vi "DFD M-Band Filter Bank Decomposition with State (Wfm).vi"(6 "state in":cluster{"state ":dbl[]}[](array[cluster]), 7 "t0":timestamp, 8 "error in (no error)":errorcluster, 9 "init?":bool, 10 "analysis bank":T1={"mBank_Filters"=[], " mBank_#Bands"=2, "mBank_ProcMethod"=enum."General", "mBank_Coeffs"=[], "mBank_Gain"=1.0, "mBank_Type"=0} {"mBank_Type" items=["Uniform", "Non-Uniform"]; "mBank_Filters"."mMRate_SumWl" min=1 max=32 step=1; "mBank_Filters"."mMRate_InputIwl" min=1 max=32 step=1; "mBank_Filters"."mMRate_GainWl" min=1 max=32 step=1; "mBank_Filters"."mMRate_OutputWl" min=1 max=32 step=1; "mBank_Filters"."mMRate_InputWl" min=1 max=32 step=1; "mBank_Filters"."mMRate_CoefWl" min=1 max=32 step=1; "mBank_Filters"."mMRate_Mode" items=["Default"=-1, "No Rate Change"=0, "Interpolation"=1, "Decimation"=2, "Interpolated"=3, "Rational"=4]}, 11 "x":waveform(dbl)={"t0"=timestamp(0 s since 1904-01-01), "dt"=0.0, "Y"=[]}) -> (0 "error out":errorcluster, 3 "M bands":waveform(dbl)[](array[waveform]), 4 "state out":cluster{"state ":dbl[]}[](array[cluster]), 5 "tf":timestamp)   [LabVIEW 2017, in "NI_DigFilter_FilterBank.lvlib"]
doc: "Filters the input waveform <B>x</B> using an M-band analysis bank specified by <B>analysis bank</B>. You must specify the most recent internal input states <B>state in</B> to get the correct output. \n\n<B>state out</B> contains the most recent internal output states, which can be used as <B>state in</B> for next call to this VI if you want to process the data continuously.\n\nYou can call the VIs in <B>Filter Bank Design</B> sub-palette to design a filter bank."
uses:
  <vilib>/addons/Digital Filter Design/NI_DigFilter_FilterBank.lvlib
  <vilib>/addons/Digital Filter Design/FilterBank.llb/Object/DFD Bank Obj.ctl
  <vilib>/addons/Digital Filter Design/_Objects.llb/DFD Multirate Filter Obj.ctl
  <vilib>/addons/Digital Filter Design/_Objects.llb/DFD Multirate Mode.ctl
  <vilib>/addons/Digital Filter Design/_Objects.llb/DFD Coef Norm Type.ctl
  <vilib>/addons/Digital Filter Design/_Objects.llb/DFD Round-off Mode.ctl
  <vilib>/addons/Digital Filter Design/_Objects.llb/DFD FXP MRate Multiply Mode.ctl
  <vilib>/addons/Digital Filter Design/FilterBank.llb/Object/DFD Filter Bank Processing Method.ctl
  <vilib>/addons/Digital Filter Design/FilterBank.llb/Object/DFD Filter Bank Type.ctl
  <vilib>/addons/Digital Filter Design/NI_DigFilterLicensed.lvlib
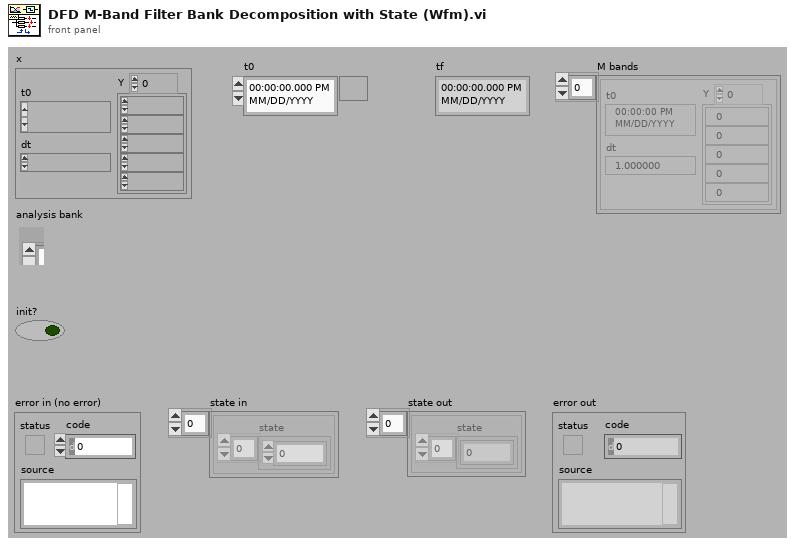
[diagram p1: front panel]
types:
  T1 = typedef "NI_DigFilter_FilterBank.lvlib/DFD Bank Obj.ctl" = cluster{"mBank_Filters":T2[], " mBank_#Bands":i32, "mBank_ProcMethod":T7, "mBank_Coeffs":dbl[], "mBank_Gain":dbl, "mBank_Type":T8}
  T2 = typedef "NI_DigFilterLicensed.lvlib/DFD Multirate Filter Obj.ctl" = cluster{"mMRate_Structure":enum16{"CIC", "FIR", "IIR", "Lattice"}, "mMRate_Mode":T3, "mMRate_Factor":i32, "mMRate_FIRParams":cluster{"mMRate_FIR_H":dbl[], "mMRate_FIR_IsNyquist?":bool, "mMRate_FIR_IsSymmetric?":bool}, "mMRate_CICParams":cluster{"mMRate_CIC_#Stage":i32, "mMRate_CIC_Lag":i32, "mMRate_CIC_Type":enum16{"Lowpass", "Highpass"}}, "mMRate_Order":i32, "mMRate_Version":string, "mMRate_Comments":string, "mMRate_RationalFactor":cluster{"mMRate_L":i32, "mMRate_M":i32}, "mMRate_Fs":dbl, "mMRate_Quantized?":bool, "mMRate_QFilterGain":dbl, "mMRate_CoefWl":i16, "mMRate_Scaling":cluster{"mMRate_ScaleByPowerOf2?":bool, "mMRate_ScaleType":T4}, "mMRate_InputWl":i16, "mMRate_OutputWl":i16, "mMRate_OutputMode":T5, "mMRate_MultMode":T6, "mMRate_BitPruning":bool, "mMRate_GainWl":i16, "mMRate_OutputFwl":i16, "mMRate_SumIwl":i16, "mMRate_InputIwl ":i16, "mMRate_SumWl":i16, "mMRate_CoefIwl":i16}
  T3 = typedef "NI_DigFilterLicensed.lvlib/DFD Multirate Mode.ctl" = i16
  T4 = typedef "NI_DigFilterLicensed.lvlib/DFD Coef Norm Type.ctl" = enum16{"No Norm", "Time Domain 1-Norm", "Time Domain 2-Norm", "Time Domain Inf-Norm"}
  T5 = typedef "NI_DigFilterLicensed.lvlib/DFD Round-off Mode.ctl" = enum16{"Nearest", "Truncation"}
  T6 = typedef "NI_DigFilterLicensed.lvlib/DFD FXP MRate Multiply Mode.ctl" = enum16{"Truncated", "Full"}
  T7 = typedef "NI_DigFilter_FilterBank.lvlib/DFD Filter Bank Processing Method.ctl" = enum16{"General", "2-Band QMF Lattice", "Cosine-Modulated"}
  T8 = typedef "NI_DigFilter_FilterBank.lvlib/DFD Filter Bank Type.ctl" = u16
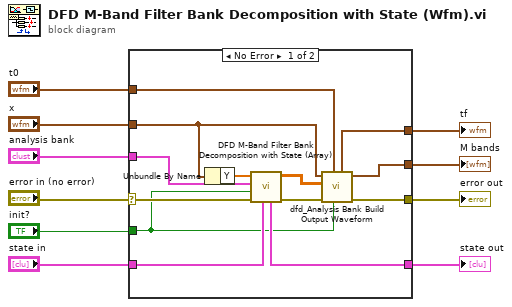
[diagram p0: block diagram]
diagram:
  n1 = case shown="No Error" "error in (no error)" {
    selector: "error in (no error)" -> [w15 w26]
    tunnel: "analysis bank" -> [w23 _]
    tunnel: [w20 _] -> w9
    tunnel: [w19 w26] -> w8
    tunnel: "state in" -> [w17 w25]
    tunnel: [w14 w25] -> w6
    tunnel: "x" -> [w16 _]
    tunnel: "init?" -> [w13 _]
    tunnel: "t0" -> [w12 w24]
    tunnel: [w11 w24] -> w1
    frame No Error {
      n2 = Unbundle By Name(w16) -> ("Y"=w18:dbl[])
      n3 = call <vilib>:"DFD M-Band Filter Bank Decomposition with State (Array).vi"("state in"=w17, "error in (no error)"=w15, "init?"=w13, "analysis bank"=w23, "M bands"=w18) -> ("error out"=w22:errorcluster, "y"=w21:dbl[][], "state out"=w14:cluster{"state ":dbl[]}[])  [unwired: 4 in]
      n4 = call <vilib>:"dfd_Analysis Bank Build Output Waveform.vi"("initH"=w13, "t0"=w12, "error in (no error)"=w22, "y"=w21, "waveform in"=w16) -> ("error out"=w19:errorcluster, "y"=w20:waveform(dbl)[], "tf"=w11:timestamp)  [unwired: 4 in]
    }
    frame Error {
    }
  }
  "error out" <- w8
  "M bands" <- w9
  "state out" <- w6
  "tf" <- w1
